vi "Editierte Zelle merken.vi"(6 "Aktion":enum16{"init", "lesen", "schreiben"}(ring), 8 "error in (no error)":errorcluster caption="Fehler (Eingang, kein Fehler)", 11 "Eingabetabelle":refnum<vi>) -> (0 "error out":errorcluster caption="Fehler (Ausgang)", 1 "Row":i32)   [LabVIEW 2020, in "Linearisierung v2.lvlib"]
uses:
  Linearisierung v2.lvlib
  Eingabetabelle.ctl
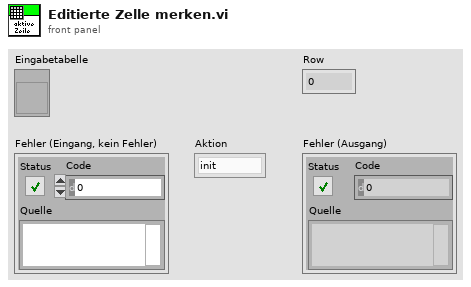
[diagram p1: front panel]
types:
  T1 = typedef "LVRowAndColumnTypeDef.ctl" = cluster{"Row":i32, "Column":i32}
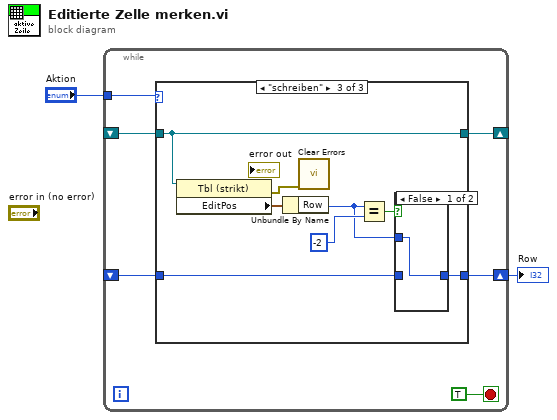
[diagram p0: block diagram]
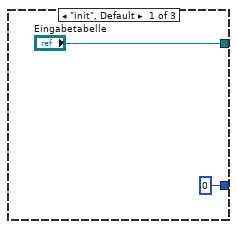
[diagram p2: hidden frame]
diagram:
  n1 = while {
    tunnel: "Aktion" -> [w7]
    shift-right: [w6] -> _
    shift-left: _ -> [w5]
    shift-right: [w4] -> w1
    shift-left: _ -> [w3]
    stop <- TRUE stop-if-true
    n2 = case shown="\"schreiben\"" w7 {
      tunnel: ["Eingabetabelle" w12 w20] -> w6
      tunnel: w5 -> [_ w12 w20]
      tunnel: [0 ("Row") w11 w14] -> w4
      tunnel: w3 -> [_ w11 w15]
      frame "init", Default {
      }
      frame "lesen" {
      }
      frame "schreiben" {
        n3 = property class="Tbl (strikt)"(reference=w20) -> (error out=w17:errorcluster, "EditPos"=w19:T1)  [unwired: 1 in, 1 out]
        n4 = Unbundle By Name(w19) -> ("Row"=w13:i32)
        n5 = call <vilib>:"Clear Errors.vi"("error in (no error)"=w17) -> ()  [unwired: 5 in, 2 out]
        n6 = Equal?(x=w13, y=-2 ("Row")) -> (x = y?=w16:bool)
        n7 = case shown="False" w16 {
          tunnel: w15 -> [_ w22]
          tunnel: [w21 w22] -> w14
          tunnel: w13 -> [w21 _]
          frame False {
          }
          frame True {
          }
        }
      }
    }
  }
  "Row" <- w1
